vi "Update VI Information.vi"(8 "error in (no error)":errorcluster, 10 "VI Infomation":T1, 11 "Model in":refnum<class "Model.lvclass">) -> (0 "error out":errorcluster, 3 "Model out":refnum<class "Model.lvclass">)   [LabVIEW 2015, in "Model.lvlib" / "Model.lvclass"]
uses:
  Model.lvclass
  Controls/VI Infomation.ctl
  Model.lvlib
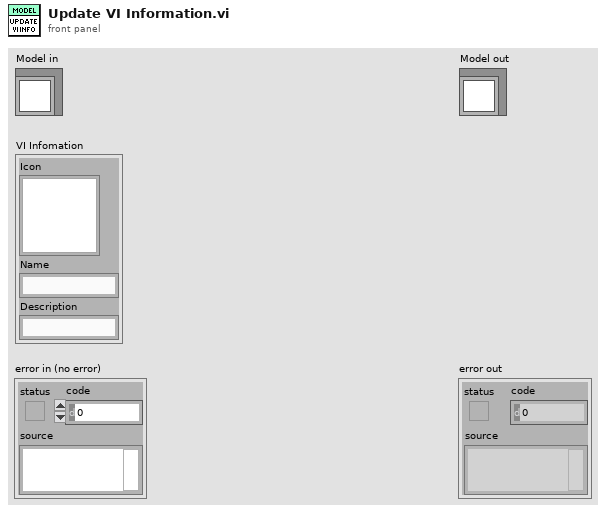
[diagram p1: front panel]
types:
  T1 = typedef "Model.lvlib/VI Infomation.ctl" = cluster{"Name":string, "Description":string, "Icon":picture}
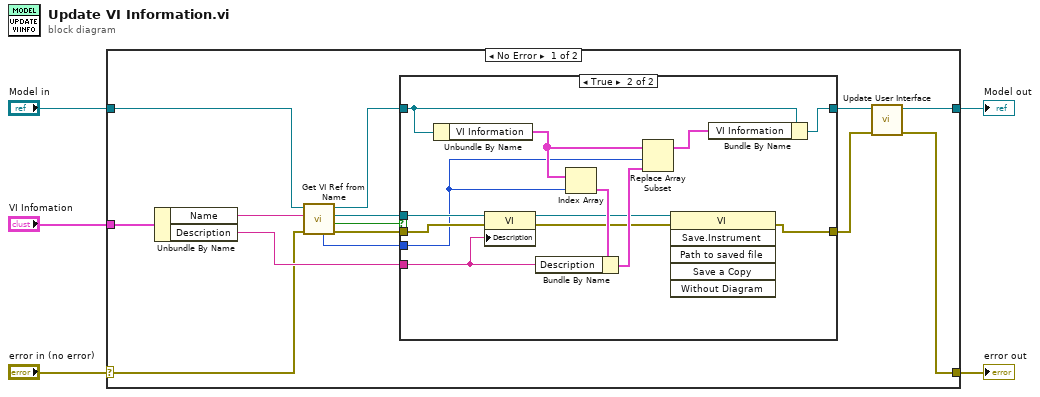
[diagram p0: block diagram]
diagram:
  n1 = case shown="No Error" "error in (no error)" {
    selector: "error in (no error)" -> [w9 w36]
    tunnel: [w11 w36] -> w4
    tunnel: [w13 w35] -> w2
    tunnel: "Model in" -> [w18 w35]
    tunnel: "VI Infomation" -> [w19 _]
    frame No Error {
      n2 = Unbundle By Name(w19) -> ("Name"=w17:string, "Description"=w14:string)
      n3 = call "Get VI Ref from Name.vi"("error in (no error)"=w9, "VI Name"=w17, "Model in"=w18) -> ("error out"=w8:errorcluster, "Found?"=w16:bool, "VI Refnum"=w15:refnum<vi>, "Model out"=w7:refnum<class "Model.lvclass">, "Index"=w10:i32)  [unwired: 4 in]
      n4 = case shown="True" w16 {
        tunnel: w15 -> [_ w34]
        tunnel: w14 -> [_ w22]
        tunnel: [w20 w23] -> w12
        tunnel: w10 -> [_ w31]
        tunnel: w8 -> [w20 w33]
        tunnel: w7 -> [w21 w28]
        tunnel: [w21 w26] -> w6
        frame False {
        }
        frame True {
          n5 = Unbundle By Name(w28) -> ("VI Information"=w32:T1[])
          n6 = property class="VI"(reference=w34, error in=w33, "Description"=w22) -> (reference out=w25:refnum<vi>, error out=w24:errorcluster)
          n7 = Index Array(array=w32, index=w31) -> (element=w30:T1)
          n8 = Bundle By Name(cluster=w30, "Description"=w22) -> (w29:T1)
          n9 = Replace Array Subset(array=w32, new element=w29, index=w31) -> (w27:T1[])
          n10 = invoke class="VI" method="Save.Instrument"(reference=w25, error in=w24) -> (error out=w23:errorcluster)  [unwired: 4 in, 5 out]
          n11 = Bundle By Name(cluster=w28, "VI Information"=w27) -> (w26:refnum<class "Model.lvclass">)
        }
      }
      n12 = call "Update User Interface.vi"("error in (no error)"=w12, "Model in"=w6) -> ("error out"=w11:errorcluster, "Model out"=w13:refnum<class "Model.lvclass">)  [unwired: 8 in]
    }
    frame Error {
    }
  }
  "error out" <- w4
  "Model out" <- w2
